vi "Init.vi"(7 "Sender":refnum<class "Sender.lvclass">, 9 "Error":errorcluster, 10 "Actor":refnum<class "Actor.lvclass">) -> (3 "Finish Msg out":refnum<class "Finish Msg.lvclass">)   [LabVIEW 2025, in "jettl.lvlib" / "Finish Msg.lvlib" / "Finish Msg.lvclass"]
uses:
  Finish Msg.lvclass
  Finish Msg.lvclass/Finish Msg.ctl
  Actor/Actor/Actor.lvclass
  Sender/Sender/Sender.lvclass
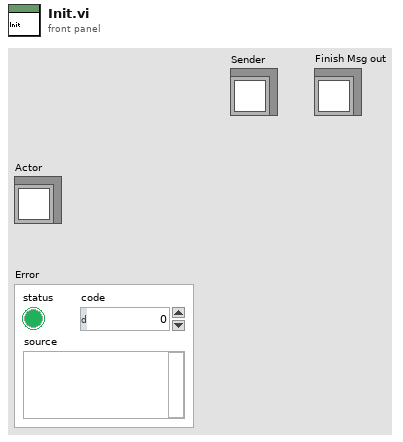
[diagram p1: front panel]
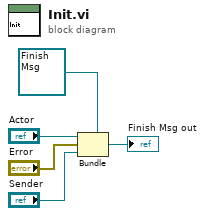
[diagram p0: block diagram]
diagram:
  n1 = Bundle "Bundle"(cluster=refnum<class "Finish Msg.lvclass"> refnum ("Last Ack Creator Queue Msg Strategy out"), "Actor", "Error", "Sender") -> (→"Finish Msg out":refnum<class "Finish Msg.lvclass">)
